vi "Subtract Offset.vi"(8 "error in (no error)":errorcluster, 9 "Offset":dbl[](array[numeric]), 10 "WFM in":waveform(dbl)[](array[waveform])) -> (0 "error out":errorcluster, 2 "WFM out":waveform(dbl)[](array[waveform]))   [LabVIEW 2016, in "Lockin.DAQ.lvclass"]
uses:
  Lockin.DAQ.lvclass
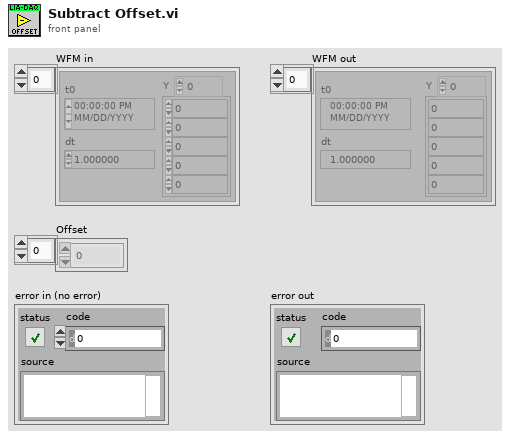
[diagram p1: front panel]
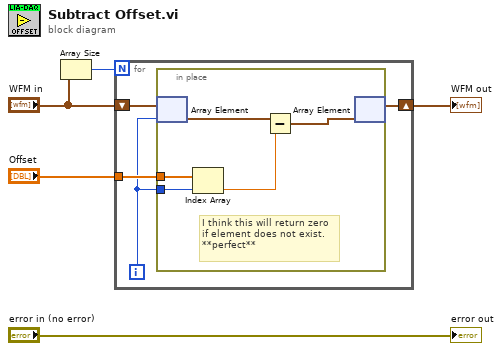
[diagram p0: block diagram]
diagram:
  n1 = Array Size(array="WFM in") -> (size(s)=w2:i32)
  n2 = for {
    N: w2 -> [_]
    tunnel: "Offset" -> [w9]
    shift-right: [w6] -> w5
    shift-left: "WFM in" -> [w7]
    i -> [w8]
    n3 = in-place {
      in-place-border: w8 -> [w14]
      in-place-border: w9 -> [w13]
      # "I think this will return zero\nif element does not exist.\n**perfect**"
      n4 = in-place-array #1(w7, w8) -> (w10:waveform(dbl))
      n5 = Index Array(array=w13, index=w14) -> (element=w12:dbl)
      n6 = Subtract(x=w10, y=w12) -> (x-y=w11:waveform(dbl))
      n7 = in-place-array #1(w11) -> (w6:waveform(dbl)[])  [unwired: 1 out]
    }
  }
  "WFM out" <- w5
  "error out" <- "error in (no error)"
